vi "CRYStepSetup Init.vi"   [LabVIEW 2013]
uses:
  CRYStepSetup Global.vi
panel:
  # "Step Init.\nconfiguration recent file and so on."
types:
  T1 = cluster{"sStepName":string, "nStepVINo":i32, "nStepVINoDisplay":i32}
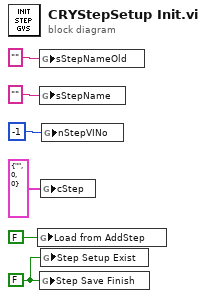
[diagram p0: block diagram]
diagram:
  w2 = FALSE ("Step Save Finish")
  n1 = global write "CRYStepSetup Global.vi" "Load from AddStep"(FALSE ("Step Setup Exist")) -> ()
  n2 = global write "CRYStepSetup Global.vi" "sStepNameOld"("" ("sStepNameOld")) -> ()
  n3 = global write "CRYStepSetup Global.vi" "sStepName"("" ("sStepName")) -> ()
  n4 = global write "CRYStepSetup Global.vi" "Step Save Finish"(w2) -> ()
  n5 = global write "CRYStepSetup Global.vi" "cStep"(T1 {"sStepName"="", "nStepVINo"=0, "nStepVINoDisplay"=0} ("cStep")) -> ()
  n6 = global write "CRYStepSetup Global.vi" "Step Setup Exist"(w2) -> ()
  n7 = global write "CRYStepSetup Global.vi" "nStepVINo"(-1 ("nStepVINo")) -> ()
